vi "echo_server.vi"() -> ()   [LabVIEW 2015]
doc: "Demonstrates how to set up a basic TCP connection, send data to the specified port once a connection has been established, and terminate the connection once the data has been sent. This VI is designed to stop if the TCP connection is terminated. The data sent in this example is an array of random numbers."
panel:
  out "String":string
  out "logs":string[][](table)
  out "name:port":string
  out "data from client":string
  in  "Client Closed":string="The client VI closed the connection."
  in  "Stop":bool
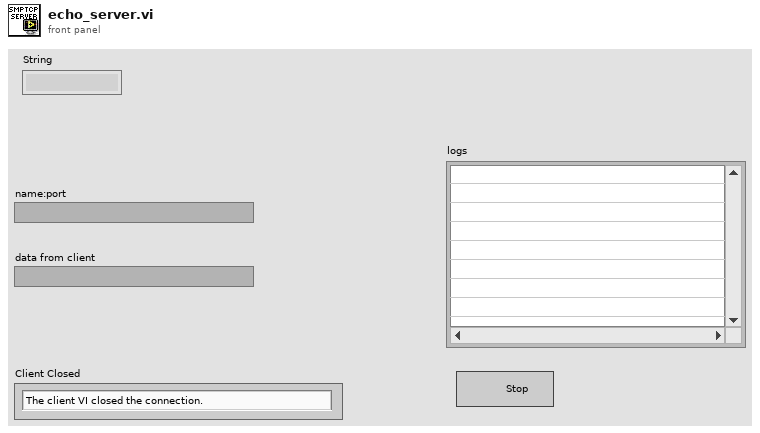
[diagram p1: front panel]
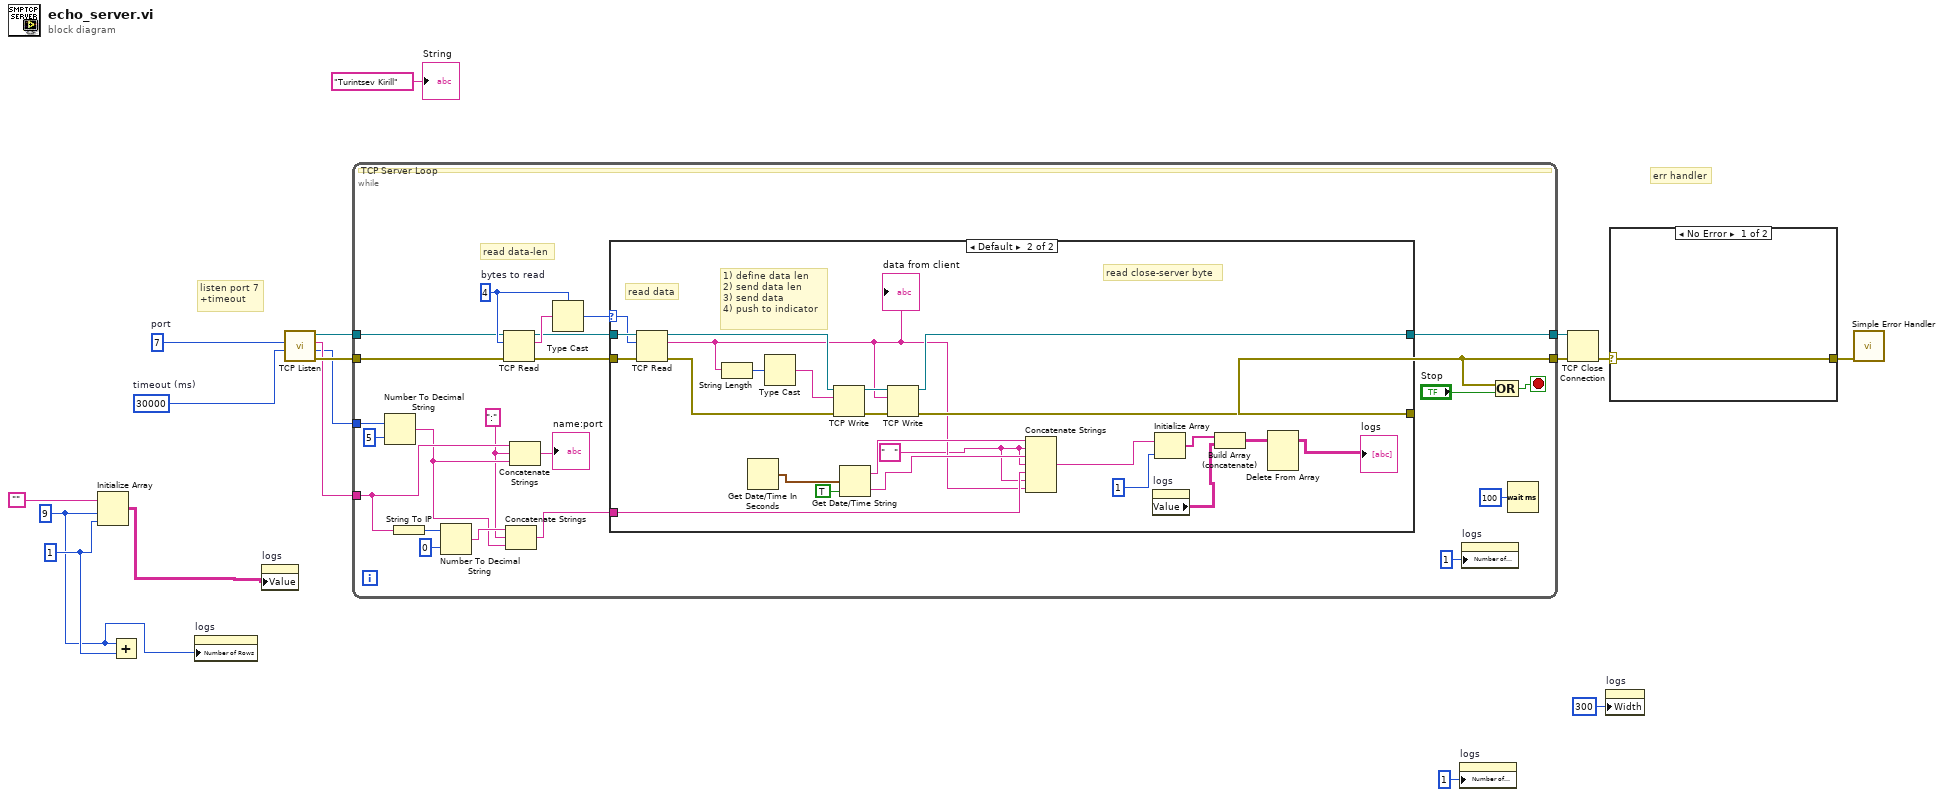
[diagram p0: block diagram]
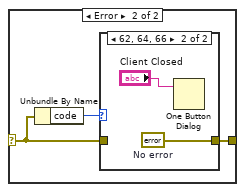
[diagram p2: hidden frame]
diagram:
  w6 = 1
  w2 = 9
  w10 = u16 7  # port
  w11 = 30000  # timeout (ms)
  # "listen port 7\n+timeout"
  # "err handler"
  n1 = Initialize Array("", w2, w6) -> (w5:string[][])
  n2 = Add(x=w2, y=w6) -> ()  [unwired: 1 out]
  n3 = property on="logs" class="Tbl (strict)"("Number of Rows"=w2) -> ()  [unwired: 2 in, 2 out]
  n4 = property on="logs" class="Tbl (strict)"("Value"=w5) -> ()  [unwired: 2 in, 2 out]
  n5 = call <vilib>:"TCP Listen.vi"("timeout ms (wait forever: -1)"=w11, "port"=w10) -> ("error out"=w12:errorcluster, "remote port"=w8:u16, "remote address"=w9:string, "connection ID"=w13:refnum<k5>)  [unwired: 5 in, 1 out]
  n6 = while {
    tunnel: [w20] -> w16
    tunnel: [w21] -> w17
    tunnel: w13 -> [w32]
    tunnel: w12 -> [w31]
    tunnel: w9 -> [w27]
    tunnel: w8 -> [w30]
    stop <- w39 stop-if-true
    w22 = ":" ("string")
    w34 = 4  # bytes to read
    # "read close-server byte"
    # "read data-len"
    # "TCP Server Loop"
    n7 = Number To Decimal String(number=w30, width (-)=i16 5) -> (decimal integer string=w23:string)
    n8 = String To IP(1:w27) -> (0:w26:u32)
    n9 = Number To Decimal String(number=w26, width (-)=i16 0) -> (decimal integer string=w24:string)
    n10 = TCP Read(connection ID=w32, bytes to read=w34, error in (no error)=w31) -> (connection ID out=w36:refnum<k5>, data out=w37:string, error out=w35:errorcluster)  [unwired: 2 in]
    n11 = Concatenate Strings(w24, w22, w23) -> (w19:string)
    n12 = Concatenate Strings(w27, w22, w23) -> (→"name:port":string)
    n13 = Type Cast(type=w34, x=w37) -> (*(type *) &x=w33:i32)
    n14 = case shown="Default" w33 {
      selector: w33 -> [_ w64]
      tunnel: w36 -> [w41 w66]
      tunnel: w35 -> [w42 w65]
      tunnel: [w41 w57] -> w21
      tunnel: [w42 w56] -> w20
      tunnel: w19 -> [_ w51]
      frame ..0 {
        # "The server has not written any data"
      }
      frame Default {
        w43 = "   " ("string")
        # "1) define data len\n2) send data len\n3) send data\n4) push to indicator"
        # "read data"
        n15 = TCP Read(connection ID=w66, bytes to read=w64, error in (no error)=w65) -> (connection ID out=w59:refnum<k5>, data out=w44:string, error out=w58:errorcluster)  [unwired: 2 in]
        "data from client" <- w44
        n16 = String Length(string=w44) -> (length=w61:i32)
        n17 = Get Date/Time In Seconds() -> (seconds since 1Jan1904=w55:timestamp)
        n18 = Type Cast(x=w61) -> (*(type *) &x=w60:string)  [unwired: 1 out]
        n19 = TCP Write(connection ID=w59, data in=w60, error in (no error)=w58) -> (connection ID out=w63:refnum<k5>, error out=w62:errorcluster)  [unwired: 2 out]
        n20 = Get Date/Time String(seconds (now)=w55, want seconds? (F)=TRUE) -> (date string=w53:string, time string=w52:string)  [unwired: 1 in]
        n21 = TCP Write(connection ID=w63, data in=w44, error in (no error)=w62) -> (connection ID out=w57:refnum<k5>, error out=w56:errorcluster)  [unwired: 2 out]
        n22 = Concatenate Strings(w53, w43, w52, w43, w51, w43, w44) -> (w50:string)
        n23 = property on="logs" class="Tbl (strict)"() -> ("Value"=w45:string[][])  [unwired: 2 in, 2 out]
        n24 = Initialize Array(w50, 1) -> (w48:string[])
        n25 = Build Array (concatenate)(w48, w45) -> (w47:string[][])
        n26 = Delete From Array(array=w47) -> (array with subset deleted=→"logs":string[][])  [unwired: 3 in, 1 out]
      }
    }
    n27 = property on="logs" class="Tbl (strict)"("Number of Columns"=u32 1) -> ()  [unwired: 2 in, 2 out]
    n28 = Compound Arithmetic op=OR(w20, "Stop") -> (w39:bool)
    n29 = Wait (ms)(milliseconds to wait=u32 100) -> ()  [unwired: 1 out]
  }
  n30 = property on="logs" class="Tbl (strict)"("Number of Columns"=u32 1) -> ()  [unwired: 2 in, 2 out]
  n31 = TCP Close Connection(connection ID=w17, error in (no error)=w16) -> (error out=w15:errorcluster)  [unwired: 2 out]
  n32 = property on="logs" class="Tbl (strict)"("Width"=u32 300 ("Size:Width")) -> ()  [unwired: 2 in, 2 out]
  n33 = case shown="No Error" w15 {
    selector: w15 -> [w67 w69]
    tunnel: [w67 w68] -> w14
    frame No Error {
    }
    frame Error {
      n34 = Unbundle By Name(w69) -> ("code"=w70:i32)
      n35 = case shown="62, 64, 66" w70 {
        tunnel: w69 -> [w71 _]
        tunnel: [w71 w73] -> w68
        frame Default {
        }
        frame 62, 64, 66 {
          w73 = errorcluster {"status"=FALSE, "code"=0, "source"=""}  # No error
          n36 = One Button Dialog(message="Client Closed") -> ()  [unwired: 1 in, 1 out]
        }
      }
    }
  }
  n37 = call <vilib>:"Simple Error Handler.vi"("error in (no error)"=w14) -> ()  [unwired: 1 in, 8 out]
  "String" <- "Turintsev Kirill" ("String")
